vi "Excel_Cell_to_RowCol.vi"(11 "Cell ([A-Z..][0-9..])":string) -> (2 "Column":i32, 3 "Row":i32)   [LabVIEW 2018]
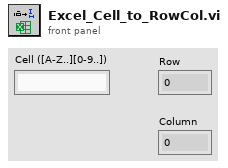
[diagram p1: front panel]
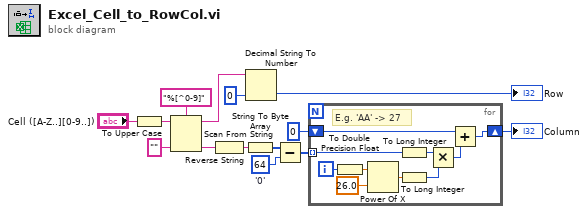
[diagram p0: block diagram]
diagram:
  w5 = u8 64  # '0'
  n1 = To Upper Case(1:"Cell ([A-Z..][0-9..])") -> (0:w13:string)
  n2 = Scan From String(format string="%[^0-9]", input string=w13, default 1="" ("default value 1")) -> (remaining string=w11:string, output 1=w7:string)  [unwired: 2 in, 2 out]
  n3 = Reverse String(1:w7) -> (0:w6:string)
  n4 = String To Byte Array(string=w6) -> (unsigned byte array=w2:u8[])
  n5 = Decimal String To Number(string=w11, default (0L)=0 ("default (0 I32)")) -> (number=→"Row":i32)  [unwired: 1 in, 1 out]
  n6 = Subtract(x=w2, y=w5) -> (x-y=w4:u8[])
  n7 = for {
    tunnel: w4 -> [w24] mode=indexing
    shift-right: [w16] -> w1
    shift-left: 0 -> [w23]
    i -> [w22]
    # "E.g. 'AA' -> 27"
    n8 = To Double Precision Float(number=w22) -> (double precision float=w21:dbl)
    n9 = Power Of X(1:26.0 ("x"), 2:w21) -> (0:w19:dbl)
    n10 = To Long Integer(number=w24) -> (32bit integer=w17:i32)
    n11 = To Long Integer(number=w19) -> (32bit integer=w18:i32)
    n12 = Multiply(x=w17, y=w18) -> (x*y=w15:i32)
    n13 = Add(x=w23, y=w15) -> (x+y=w16:i32)
  }
  "Column" <- w1
